vi "VernierStableTest.vi"(8 "error in (no error)":errorcluster, 9 "Custard":dbl(slide) scale=0.0..50.0, 10 "Time Target (s)":dbl=1.0, 11 "i":u32) -> (0 "error out":errorcluster, 2 "Time has Elapsed":bool)   [LabVIEW 2019, in "Vernier.lvlib"]
uses:
  Vernier.lvlib
panel:
  out ".not. x?":bool
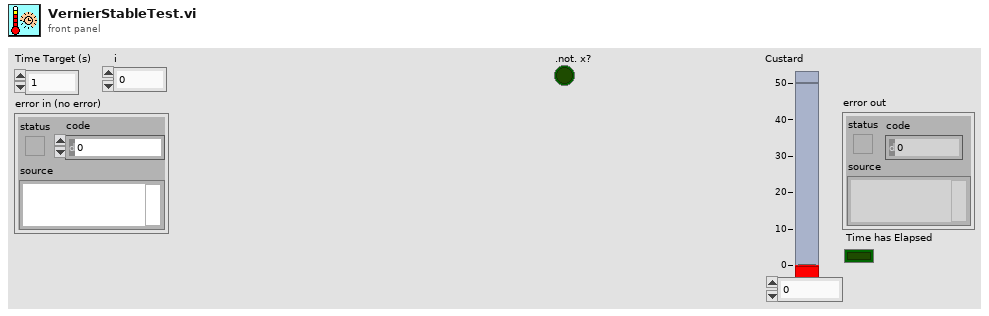
[diagram p1: front panel]
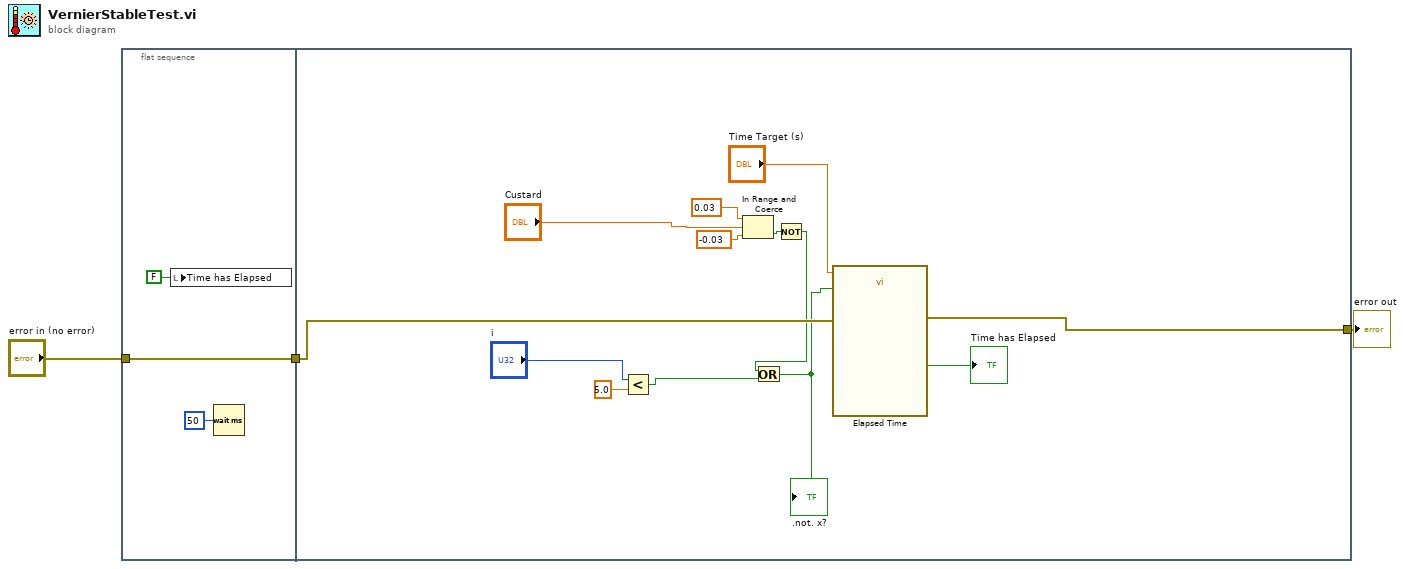
[diagram p0: block diagram]
diagram:
  n1 = flat-sequence {
    tunnel: "error in (no error)" -> [w6]
    tunnel: [w6] -> w1
    tunnel: [w18] -> w2
    tunnel: w1 -> [w19]
    frame #0 {
      n2 = local write "Time has Elapsed"(FALSE ("Time has Elapsed")) -> ()
      n3 = Wait (ms)(milliseconds to wait=u32 50) -> ()  [unwired: 1 out]
    }
    frame #1 {
      n4 = Less?(x="i", y=5.0) -> (x < y?=w8:bool)
      n5 = In Range and Coerce(upper limit=0.03, x="Custard", lower limit=-0.03) -> (In Range?=w15:bool)  [unwired: 1 out]
      n6 = Not(x=w15) -> (.not. x?=w11:bool)
      n7 = Or(x=w11, y=w8) -> (x .or. y?=w10:bool)
      ".not. x?" <- w10
      n8 = call "Elapsed Time"("Time Target (s)"="Time Target (s)", "Reset"=w10, "error in (no error)"=w19) -> ("Time has Elapsed"=→"Time has Elapsed":bool, "error out"=w18:errorcluster)  [unwired: 9 in, 6 out]
    }
  }
  "error out" <- w2
